vi "Set Fault Msg.vi"(8 "error in":errorcluster, 10 "Sequence Context":refnum<k7>, 11 "FaultCode":i32=6144) -> (0 "error out":errorcluster, 2 "Fault codes":cluster{"Bit":string, "Description":string}[](array[cluster]), 3 "PLC Fault":bool caption="Fault")   [LabVIEW 2021, in "OPCUA.lvlib"]
uses:
  OPCUA.lvlib
  <vilib>/addons/TestStand/_TSUtility.llb/TestStand - Get Property Value (Number {Signed 32-bit Integer}).vi
panel:
  # "Bit"
  # "Fault"
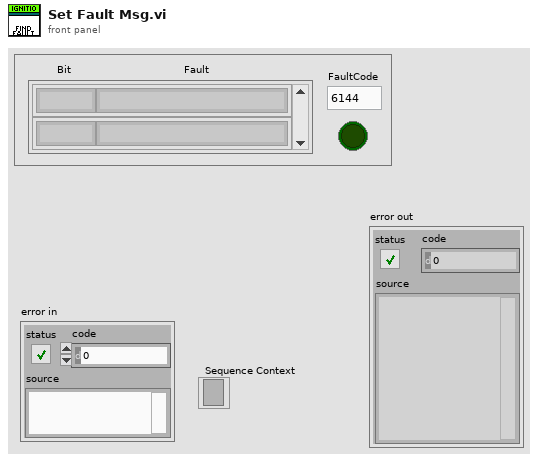
[diagram p1: front panel]
types:
  T1 = enum32{"Invalid", "Standard", "Closed", "Hidden", "Minimized", "Maximized"}
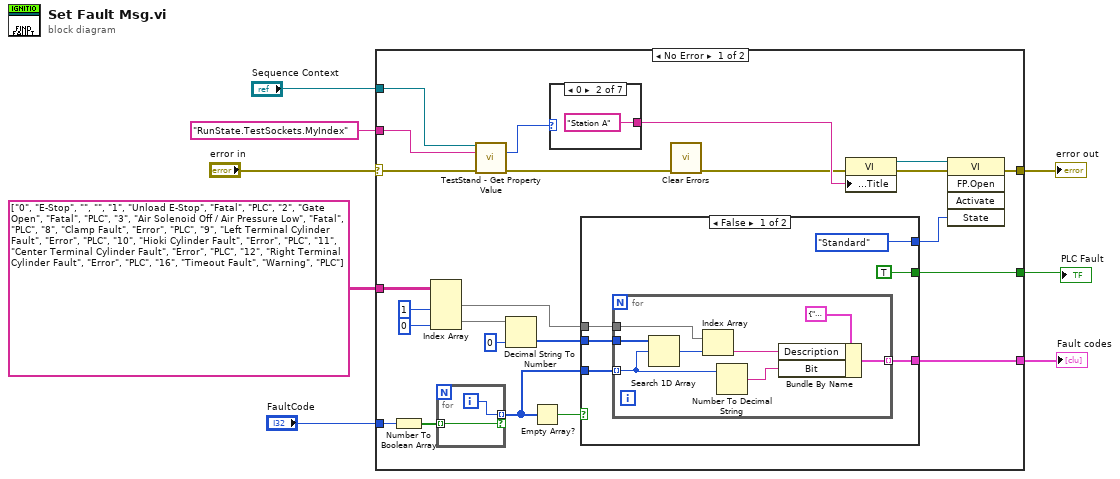
[diagram p0: block diagram]
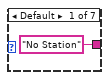
[diagram p2: hidden frame]
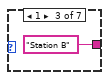
[diagram p3: hidden frame]
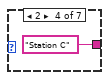
[diagram p4: hidden frame]
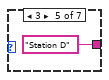
[diagram p5: hidden frame]
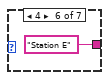
[diagram p6: hidden frame]
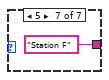
[diagram p7: hidden frame]
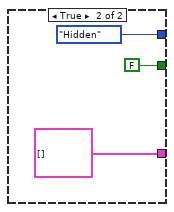
[diagram p8: hidden frame]
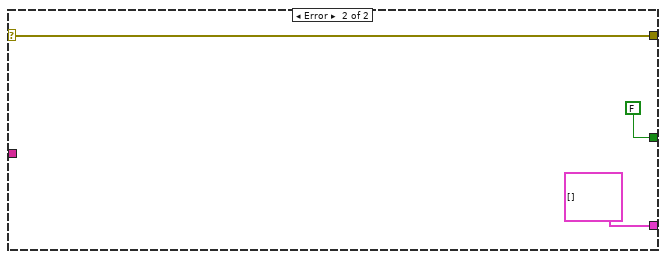
[diagram p9: hidden frame]
diagram:
  n1 = case shown="No Error" "error in" {
    selector: "error in" -> [w31 w61]
    tunnel: string[][] [["0", "E-Stop", "", ""], ["1", "Unload E-Stop", "Fatal", "PLC"], ["2", "Gate Open", "Fatal", "PLC"], ["3", "Air Solenoid Off / Air Pressure Low", "Fatal", "PLC"], ["8", "Clamp Fault", "Error", "PLC"], ["9", "Left Terminal Cylinder Fault", "Error", "PLC"], ["10", "Hioki Cylinder Fault", "Error", "PLC"], ["11", "Center Terminal Cylinder Fault", "Error", "PLC"], ["12", "Right Terminal Cylinder Fault", "Error", "PLC"], ["16", "Timeout Fault", "Warning", "PLC"]] -> [w18 _]
    tunnel: "FaultCode" -> [w20 _]
    tunnel: [w23 w61] -> w7
    tunnel: "Sequence Context" -> [w32 _]
    tunnel: "RunState.TestSockets.MyIndex" ("Lookup String") -> [w29 _]
    tunnel: [w13 cluster{"Bit":string, "Description":string}[] []] -> w2
    tunnel: [w9 FALSE] -> w1
    frame No Error {
      n2 = Number To Boolean Array(number=w20) -> (Boolean array=w19:bool[])
      n3 = Index Array(array=w18, index (col) #1=1 ("disabled index (col)"), index (col) #2=0 ("index (col)")) -> (element #1=w10:string[], element #2=w11:string[])  [unwired: 2 in]
      n4 = for {
        tunnel: w19 -> [w57] mode=indexing
        tunnel: [w58] -> w12 mode=indexing if=w57
        i -> [w58]
      }
      n5 = call-poly <vilib>:"TestStand - Get Property Value.vi"("Sequence Context In"=w32, "Lookup String"=w29, "error in (no error)"=w31) -> ("Value"=w30:i32, "error out"=w28:errorcluster)  [unwired: 10 in, 1 out]
      n6 = Decimal String To Number(string=w11, default (0L)=0 ("default (0 I32)")) -> (number=w14:i32[])  [unwired: 1 in, 1 out]
      n7 = Empty Array?(array=w12) -> (empty?=w16:bool)
      n8 = case shown="0" w30 {
        tunnel: ["No Station" ("initial string") "Station A" ("initial string") "Station B" ("initial string") "Station C" ("initial string") "Station D" ("initial string") "Station E" ("initial string") "Station F" ("initial string")] -> w27
        frame Default {
        }
        frame 0 {
        }
        frame 1 {
        }
        frame 2 {
        }
        frame 3 {
        }
        frame 4 {
        }
        frame 5 {
        }
      }
      n9 = case shown="False" w16 {
        tunnel: [T1."Standard" ("State") T1."Hidden" ("State")] -> w15
        tunnel: [w41 cluster{"Bit":string, "Description":string}[] []] -> w13
        tunnel: [TRUE FALSE] -> w9
        tunnel: w14 -> [w44 _]
        tunnel: w12 -> [w43 _]
        tunnel: w10 -> [w42 _]
        frame False {
          n10 = for {
            tunnel: w43 -> [w48] mode=indexing
            tunnel: w44 -> [w53]
            tunnel: w42 -> [w51]
            tunnel: [w47] -> w41 mode=indexing
            n11 = Search 1D Array(1D array=w53, element=w48) -> (index of element=w52:i32)  [unwired: 1 in]
            n12 = Index Array(array=w51, index=w52) -> (element=w49:string)
            n13 = Number To Decimal String(number=w48) -> (decimal integer string=w46:string)  [unwired: 1 in]
            n14 = Bundle By Name(cluster=cluster{"Bit":string, "Description":string} {"Bit"="", "Description"=""} ("Fault"), "Description"=w49, "Bit"=w46) -> (w47:cluster{"Bit":string, "Description":string})
          }
        }
        frame True {
        }
      }
      n15 = call <vilib>:"Clear Errors.vi"("error in (no error)"=w28) -> ("error out"=w24:errorcluster)  [unwired: 5 in, 1 out]
      n16 = property class="VI"(error in=w24, "Front Panel.Title"=w27) -> (reference out=w25:refnum<vi>, error out=w26:errorcluster)  [unwired: 1 in]
      n17 = invoke class="VI" method="FP.Open"(reference=w25, error in=w26, "State"=w15) -> (error out=w23:errorcluster)  [unwired: 2 in, 4 out]
    }
    frame Error {
    }
  }
  "error out" <- w7
  "Fault codes" <- w2
  "PLC Fault" <- w1
